vi "Drag Start (inline).vi"(8 "error in (no error)":errorcluster, 11 "BetterHandle in":refnum<class "BetterHandle.lvclass">) -> (0 "error out":errorcluster, 2 "BetterDropOp":refnum<class "BetterDropOp.lvclass">, 3 "BetterHandle out":refnum<class "BetterHandle.lvclass">)   [LabVIEW 2020, in "BetterDragAndDrop.lvlib" / "BetterHandle.lvclass"]
uses:
  BetterHandle.lvclass
  BetterDropOp/BetterDropOp.lvclass
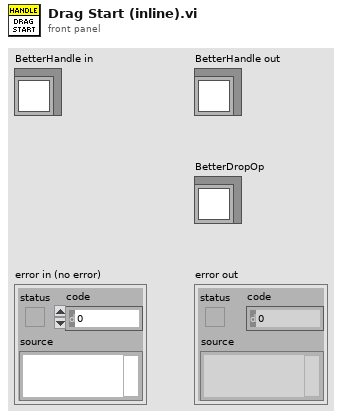
[diagram p1: front panel]
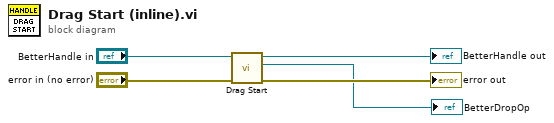
[diagram p0: block diagram]
diagram:
  n1 = call-dynamic "Drag Start.vi"("error in (no error)"="error in (no error)", "BetterHandle in"="BetterHandle in") -> ("error out"=→"error out":errorcluster, "BetterDropOp"=→"BetterDropOp":refnum<class "BetterDropOp.lvclass">, "BetterHandle out"=→"BetterHandle out":refnum<class "BetterHandle.lvclass">)  [unwired: 7 in]
